vi "Serialize Core.vi"(8 "error in (no error)":errorcluster, 11 "Serializable Message in":refnum<class "echo Msg.lvclass">) -> (0 "error out":errorcluster, 2 "Serialized Message":string)   [LabVIEW 2020, in "Chat Window.lvlib" / "echo Msg.lvclass"]
uses:
  echo Msg.lvclass
  echo Msg.lvclass/echo Msg.ctl
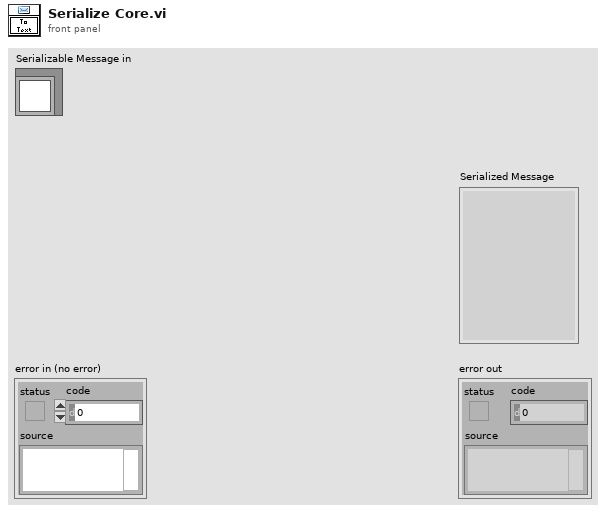
[diagram p1: front panel]
types:
  T1 = cluster{"Message":string, "id":string, "exec_time":i32}
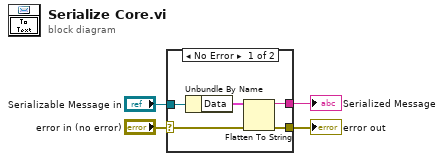
[diagram p0: block diagram]
diagram:
  n1 = case shown="No Error" "error in (no error)" {
    selector: "error in (no error)" -> [w7 w10]
    tunnel: [w5 w10] -> w3
    tunnel: "Serializable Message in" -> [w9 _]
    tunnel: [w6 _] -> w1
    frame No Error {
      n2 = Unbundle By Name(w9) -> ("Data"=w8:T1)
      n3 = Flatten To String(anything=w8, error in (no error)=w7) -> (data string=w6:string, error out=w5:errorcluster)  [unwired: 2 in, 1 out]
    }
    frame Error {
    }
  }
  "error out" <- w3
  "Serialized Message" <- w1
